vi "tvac_gui_v1.vi"() -> ()   [LabVIEW 2017]
uses:
  <vilib>/httpClient/ClientHandle.ctl
  <vilib>/httpClient/POSTBuffer.vi
  <vilib>/httpClient/LabVIEWHTTPClient.lvlib
panel:
  out "body 2":string
  in  "Tab Control":T1(tab)
  in  "TC Graph 2":T2
  out "TC Display":T3
  out "Waveform Chart":waveform(dbl)[](graph)=[{"t0"=timestamp(3580757854.087 s since 1904-01-01), "dt"=1.0, "Y"=[750.0616827041697]}, {"t0"=timestamp(3580757854.087 s since 1904-01-01), "dt"=1.0, "Y"=[750.0616827041697]}, {"t0"=timestamp(3580757854.087 s since 1904-01-01), "dt"=1.0, "Y"=[750.0616827041697]}]
  out "body":string
  in  "stop":bool
  in  "Run 4":bool
  in  "Run 3":bool
  in  "Run 2":bool
  in  "Run":bool
  in  "Zone 1":T4 {"average" items=["Average", "Maximum", "Minimum"]}
  out "body 3":string
  out "JSON string":string
  out "Custom Graphs 4":dbl[](graph)
  out "Custom Graphs 3":dbl[](graph)
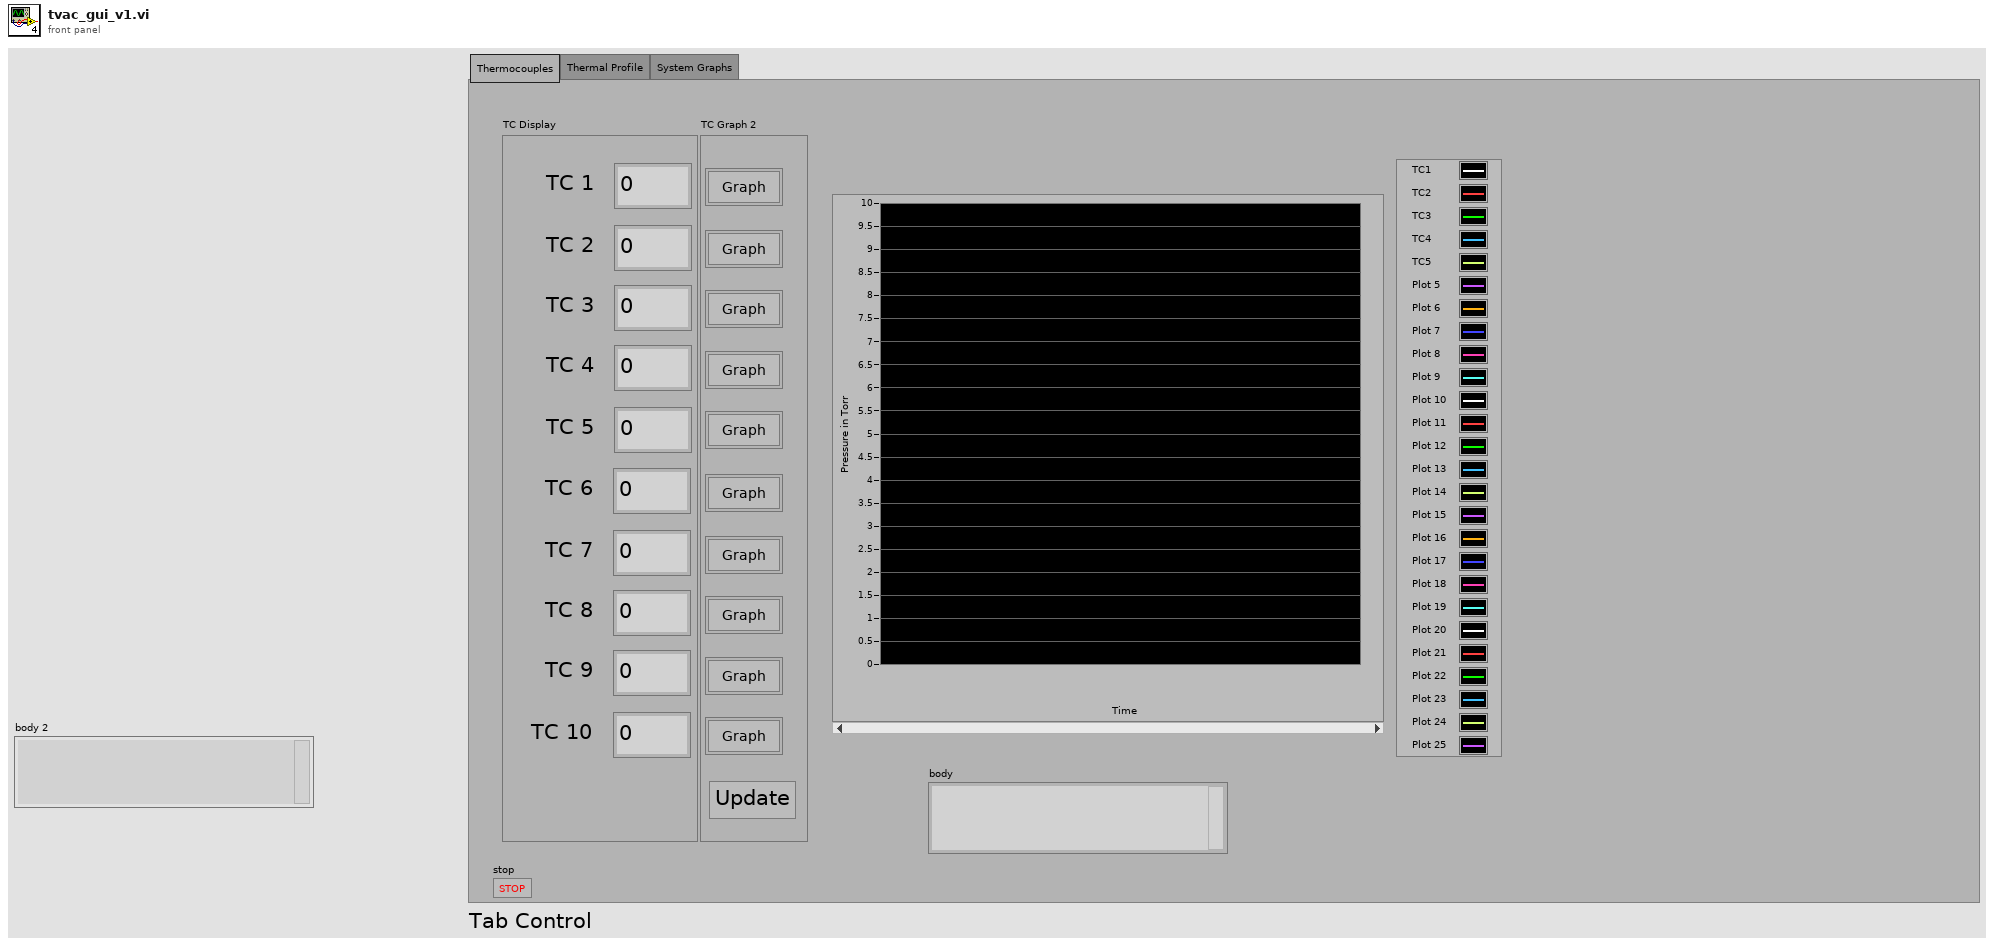
[diagram p1: front panel]
types:
  T1 = enum32{"Thermocouples", "Thermal Profile", "System Graphs"}
  T2 = cluster{"TC 1":bool, "TC 2":bool, "TC 3":bool, "TC 4":bool, "TC 5":bool, "TC 6":bool, "TC 7":bool, "TC 8":bool, "TC 9":bool, "TC 10":bool, "Update":bool}
  T3 = cluster{"TC 1":dbl, "TC 2":dbl, "TC 3":dbl, "TC 4":dbl, "TC 5":dbl, "TC 6":dbl, "TC 7":dbl, "TC 8":dbl, "TC 9":dbl, "TC 10":dbl}
  T4 = cluster{"zone":dbl, "average":u16, "thermocouples":dbl[], "thermalprofile":cluster{"thermalsetpoint":dbl, "tempgoal":dbl, "ramp":dbl, "soakduration":dbl}}
  T5 = typedef "LabVIEWHTTPClient.lvlib/ClientHandle.ctl" = refnum<k1>
  T6 = cluster{"go":bool, "Http session":T5, "URL prefex":string}
  T7 = cluster{"time":string, "tcs":cluster{"thermocouple":i32, "time":i32, "temp":i32, "working":i32}[]}
  T8 = cluster{"thermocouple":i32, "time":i32, "temp":i32, "working":i32}[]
  T9 = cluster{"thermocouple":i32, "time":i32, "temp":i32, "working":i32}
  T10 = cluster{"zone":i32, "profileuuid":string, "average":i32, "zoneUUID":string, "termalprofiles":cluster{"termalsetpoint":i32, "tempgoal":i32, "temp":i32, "soakduration":i32, "duration":i32, "ramp":i32}[], "thermocouples":cluster{"thermocouple":i32, "time":i32, "temp":i32, "working":string}[]}
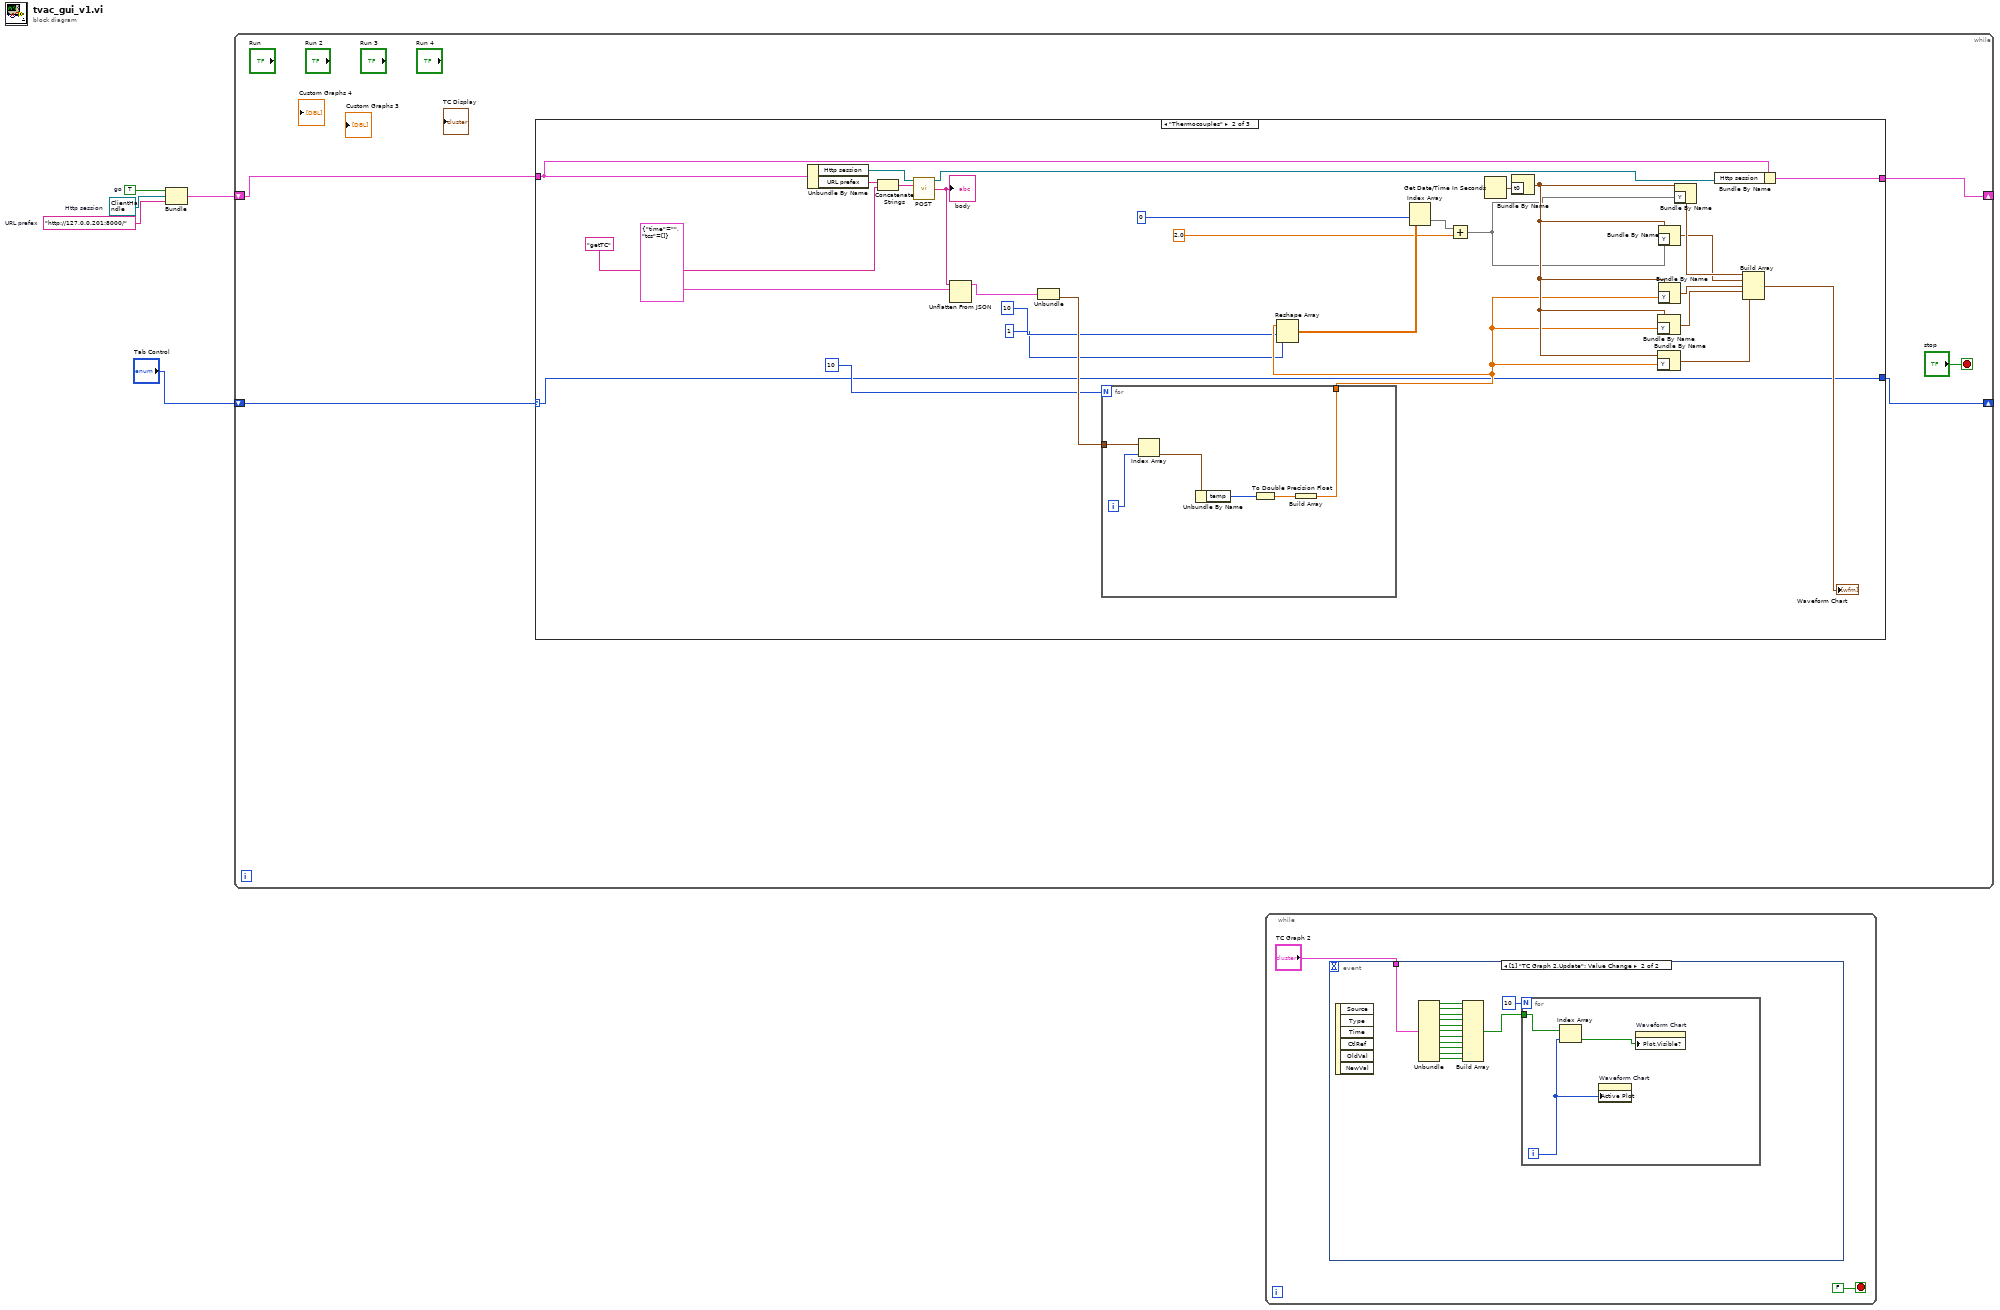
[diagram p0: block diagram]
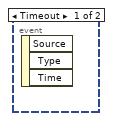
[diagram p2: hidden frame]
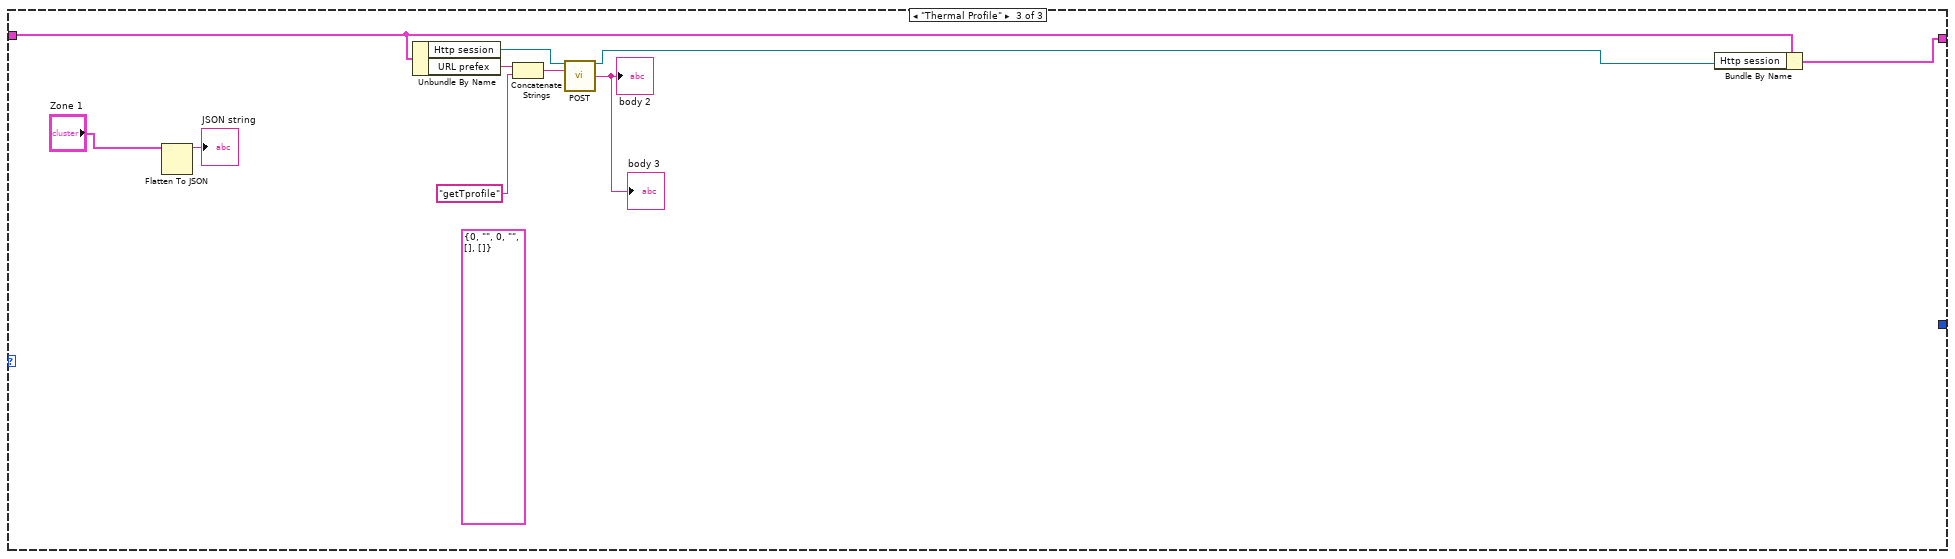
[diagram p4: hidden frame]
diagram:
  w3 = "http://127.0.0.201:8000/"  # URL prefex
  w4 = T5 refnum  # Http session
  w5 = TRUE  # go
  n1 = Bundle("go"=w5, "Http session"=w4, "URL prefex"=w3) -> (w2:T6)  [unwired: 1 in]
  n2 = while {
    shift-right: [w9] -> _
    shift-left: w2 -> [w10]
    shift-right: [w7] -> _
    shift-left: "Tab Control" -> [w8]
    stop <- "stop" stop-if-true
    n3 = case shown="\"Thermocouples\"" w8 {
      selector: w8 -> [_ w11 _]
      tunnel: w10 -> [_ w23 w48]
      tunnel: [_ w22 w49] -> w9
      tunnel: [_ w11 _] -> w7
      frame "System Graphs" {
      }
      frame "Thermocouples" {
        n4 = Unbundle By Name(w23) -> ("Http session"=w31:T5, "URL prefex"=w29:string)
        n5 = Concatenate Strings(w29, "getTC" ("url")) -> (w30:string)
        n6 = call-poly <vilib>:"POST.vi"("client handle"=w31, "url"=w30) -> ("client handle out"=w24:T5, "body"=w26:string)  [unwired: 10 in, 2 out]
        "body" <- w26
        n7 = Unflatten From JSON(JSON string=w26, type and defaults=T7 {"time"="", "tcs"=[]}) -> (value=w25:T7)  [unwired: 5 in, 1 out]
        n8 = Unbundle(w25) -> ("tcs"=w21:T8)  [unwired: 1 out]
        n9 = for {
          N: 10 -> [_]
          tunnel: w21 -> [w45]
          tunnel: [w40] -> w19
          i -> [w44]
          n10 = Index Array(array=w45, index=w44) -> (element=w43:T9)
          n11 = Unbundle By Name(w43) -> ("temp"=w42:i32)
          n12 = To Double Precision Float(number=w42) -> (double precision float=w41:dbl)
          n13 = Build Array(w41) -> (w40:dbl[])
        }
        n14 = Reshape Array(w19, 10 ("dimension size"), 1 ("dimension size")) -> (w16:dbl[][])
        n15 = Index Array(array=w16, index (row)=0) -> (element=w13:dbl[])  [unwired: 1 in]
        n16 = Add(x=w13, y=2.0) -> (x+y=w12:dbl[])
        n17 = Get Date/Time In Seconds() -> (seconds since 1Jan1904=w39:timestamp)
        n18 = Bundle By Name("t0"=w39) -> (w32:waveform(dbl))  [unwired: 1 in]
        n19 = Bundle By Name(cluster=w32, "Y"=w19) -> (w34:waveform(dbl))
        n20 = Bundle By Name(cluster=w32, "Y"=w19) -> (w33:waveform(dbl))
        n21 = Bundle By Name(cluster=w32, "Y"=w12) -> (w37:waveform(dbl))
        n22 = Bundle By Name(cluster=w32, "Y"=w19) -> (w36:waveform(dbl))
        n23 = Bundle By Name(cluster=w32, "Y"=w12) -> (w38:waveform(dbl))
        n24 = Bundle By Name(cluster=w23, "Http session"=w24) -> (w22:T6)
        n25 = Build Array(w38, w37, w36, w34, w33) -> (→"Waveform Chart":waveform(dbl)[])
      }
      frame "Thermal Profile" {
        (unwired) T10 {"zone"=0, "profileuuid"="", "average"=0, "zoneUUID"="", "termalprofiles"=[], "thermocouples"=[]}
        n26 = Flatten To JSON(anything="Zone 1") -> (JSON string=→"JSON string":string)  [unwired: 2 in, 1 out]
        n27 = Unbundle By Name(w48) -> ("Http session"=w55:T5, "URL prefex"=w53:string)
        n28 = Concatenate Strings(w53, "getTprofile" ("url")) -> (w54:string)
        n29 = call-poly <vilib>:"POST.vi"("client handle"=w55, "url"=w54) -> ("client handle out"=w50:T5, "body"=→"body 2" →"body 3":string)  [unwired: 10 in, 2 out]
        n30 = Bundle By Name(cluster=w48, "Http session"=w50) -> (w49:T6)
      }
    }
  }
  n31 = while {
    stop <- FALSE stop-if-true
    n32 = event shown="[1] \"TC Graph 2.Update\": Value Change" {
      selector: _ -> [_ _]
      dyn-events: _ -> [_ _]
      timeout: _ -> [_ _]
      tunnel: "TC Graph 2" -> [_ w71]
      event Timeout {
        n33 = event-data() -> ()  [unwired: 1 in, 3 out]
      }
      event "TC Graph 2.Update": Value Change {
        n34 = event-data() -> ()  [unwired: 1 in, 6 out]
        n35 = Unbundle(w71) -> ("TC 1"=w70:bool, "TC 2"=w69:bool, "TC 3"=w68:bool, "TC 4"=w67:bool, "TC 5"=w66:bool, "TC 6"=w63:bool, "TC 7"=w62:bool, "TC 8"=w61:bool, "TC 9"=w60:bool, "TC 10"=w59:bool, "Update"=w58:bool)
        n36 = Build Array(w70, w69, w68, w67, w66, w63, w62, w61, w60, w59, w58) -> (w65:bool[])
        n37 = for {
          N: 10 -> [_]
          tunnel: w65 -> [w74]
          i -> [w73]
          n38 = Index Array(array=w74, index=w73) -> (element=w72:bool)
          n39 = property on="Waveform Chart" class="WFChart (strict)"("Active Plot"=w73) -> ()  [unwired: 2 in, 2 out]
          n40 = property on="Waveform Chart" class="WFChart (strict)"("Plot.Visible?"=w72) -> ()  [unwired: 2 in, 2 out]
        }
      }
    }
  }
